vi "piezoUSBWrite.vi"(1 "mode":u16(ring) items=["fractional", "voltage (V)", "position (um)"], 2 "position":dbl) -> ()   [LabVIEW 2017]
uses:
  globalDevices.vi
  Piezo/lvlib/Madlib.lvlib
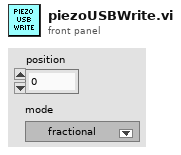
[diagram p1: front panel]
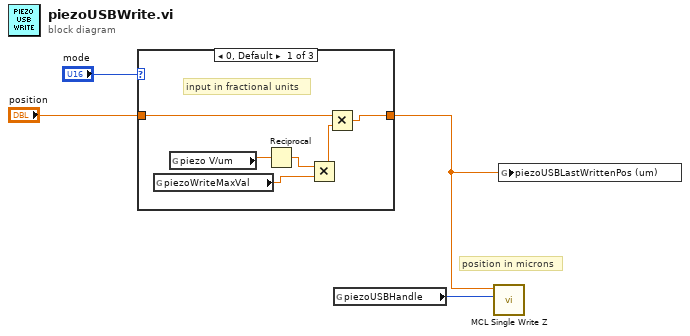
[diagram p0: block diagram]
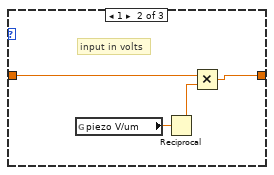
[diagram p2: hidden frame]
diagram:
  # "position in microns"
  n1 = case shown="0, Default" "mode" {
    tunnel: "position" -> [w10 w14 w15]
    tunnel: [w9 w13 w15] -> w1
    frame 0, Default {
      # "input in fractional units"
      n2 = global read "globalDevices.vi" "piezoWriteMaxVal"() -> (w8:dbl)
      n3 = global read "globalDevices.vi" "piezo V/um"() -> (w7:dbl)
      n4 = Reciprocal(x=w7) -> (1/x=w6:dbl)
      n5 = Multiply(x=w6, y=w8) -> (x*y=w5:dbl)
      n6 = Multiply(x=w10, y=w5) -> (x*y=w9:dbl)
    }
    frame 1 {
      # "input in volts"
      n7 = global read "globalDevices.vi" "piezo V/um"() -> (w12:dbl)
      n8 = Reciprocal(x=w12) -> (1/x=w11:dbl)
      n9 = Multiply(x=w14, y=w11) -> (x*y=w13:dbl)
    }
    frame 2 {
      # "input in microns"
    }
  }
  n10 = global read "globalDevices.vi" "piezoUSBHandle"() -> (w4:i32)
  n11 = call "MCL Single Write Z.vi"("handle"=w4, "position"=w1) -> ()  [unwired: 9 in, 1 out]
  n12 = global write "globalDevices.vi" "piezoUSBLastWrittenPos (um)"(w1) -> ()
